vi "Self-Test.vi"(8 "error in (no error)":errorcluster {"code" format="%.0x"}, 11 "VISA Resource Name":refnum<visa-resource-name>) -> (0 "error out":errorcluster {"code" format="%.0x"}, 1 "Self-Test Response":string, 2 "Self-Test Error":u32, 3 "VISA Resource Name Out":refnum<visa-resource-name>)   [LabVIEW 2011, in "Agilent 546XX Series.lvlib"]
doc: "This VI resets the instrument to a known state and sends initialization commands to the instrument. The initialization commands set instrument settings such as Headers Off, Short Command form, and Data Transfer Binary to the state necessary for the operation of the instrument driver."
uses:
  Agilent 546XX Series.lvlib
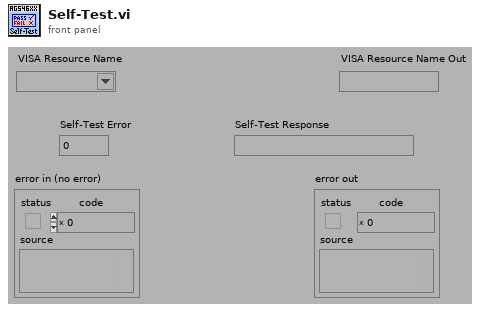
[diagram p1: front panel]
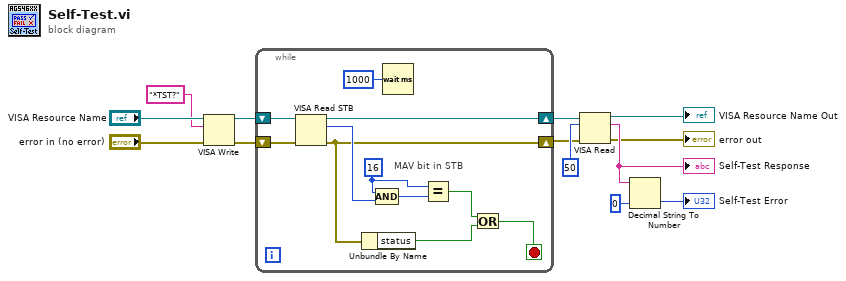
[diagram p0: block diagram]
diagram:
  n1 = VISA Write(VISA resource name="VISA Resource Name", write buffer="*TST?", error in (no error)="error in (no error)") -> (VISA resource name out=w5:refnum<visa-resource-name>, error out=w4:errorcluster)  [unwired: 1 out]
  n2 = while {
    shift-right: [w17] -> w6
    shift-left: w4 -> [w21]
    shift-right: [w19] -> w7
    shift-left: w5 -> [w20]
    stop <- w14 stop-if-true
    w24 = u16 16 ("value")
    # "MAV bit in STB"
    n3 = VISA Read STB(8:w21, 11:w20) -> (0:w17:errorcluster, 2:w22:u16, 3:w19:refnum<visa-resource-name>)
    n4 = Unbundle By Name(w17) -> ("status"=w15:bool)
    n5 = Compound Arithmetic op=AND(w24, w22) -> (w23:u16)
    n6 = Wait (ms)(milliseconds to wait=u32 1000) -> ()  [unwired: 1 out]
    n7 = Equal?(x=w24, y=w23) -> (x = y?=w16:bool)
    n8 = Or(x=w16, y=w15) -> (x .or. y?=w14:bool)
  }
  n9 = VISA Read(VISA resource name=w7, byte count=u32 50, error in (no error)=w6) -> (VISA resource name out=→"VISA Resource Name Out":refnum<visa-resource-name>, read buffer=w10:string, error out=→"error out":errorcluster)  [unwired: 1 out]
  "Self-Test Response" <- w10
  n10 = Decimal String To Number(string=w10, default (0L)=u32 0 ("Default (0L)")) -> (number=→"Self-Test Error":u32)  [unwired: 1 in, 1 out]
